vi "Pressure_2_R1.vi"() -> ()   [LabVIEW 2020]
uses:
  Support/Controls/Cmd_Mouse Popup.ctl
  Support/Controls/Clst_Initialize Input.ctl
  Support/Controls/Cmd_Var Data IO.ctl
  Variables/Global_Cal Info.vi
panel:
  in  "Measured_ADJ":string[][](table) caption="Measured (조정후)"
  in  "입력전압":dbl=10.0 caption="(V)"
  in  "정격출력":dbl
  in  "최소출력":dbl
  in  "출력단위":string(combo)="V"
  out "최소용량":string
  out "분동조합":string[][](table)
  out "Form":string[][](table)
  in  "교정방법":string(combo)="기본교정"
  out "Resolution":string[][](table) caption="Spec"
  in  "Spec 변경":bool
  in  "Random":bool
  out "Spec":string[][](table)
  out "제목":string
  out "에러 출력":errorcluster
  out "Condition":string[][](table)
  out "최소눈금":string
  out "단위":string
  out "최대용량":string
  in  "Measured":string[][](table)
  out "Load?":bool
  # "※ 압력기준기 복수 선택 시 분동식 압력계\n    우선 적용됨."
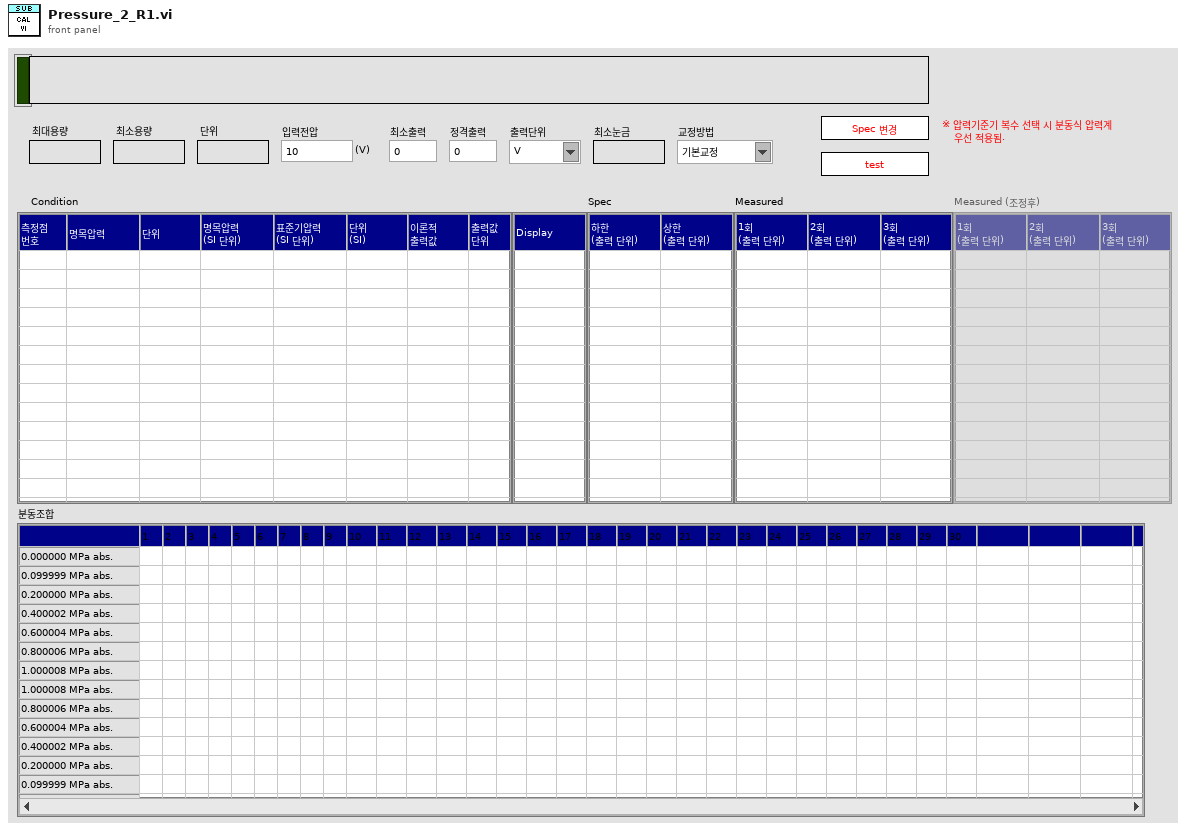
[diagram p1: front panel]
types:
  T1 = typedef "Cmd_Mouse Popup.ctl" = enum16{"활성화", "메뉴선택"}
  T2 = cluster{"Shift":bool, "Ctrl":bool, "Alt":bool, "Cmd":bool, "Opt":bool}
  T3 = typedef "Clst_Initialize Input.ctl" = cluster{"Initialize 1":cluster{"Condition":refnum<vi>[], "Spec":refnum<vi>[], "Measured":refnum<vi>[], "Resolution":refnum<vi>[], "Func_ext":string, "제목":refnum<vi>, "Measured_ADJ":refnum<vi>[]}, "Initialize 2":cluster{"문자열":refnum<vi>[], "콤보박스":refnum<vi>[], "링":refnum<vi>[], "열거형":refnum<vi>[], "테이블":refnum<vi>[], "여러열":refnum<vi>[], "디지털(DBL)":refnum<vi>[], "3D string":refnum<vi>[], "ctrl":refnum<vi>[], "boolean":refnum<vi>[]}}
  T4 = typedef "Cmd_Var Data IO.ctl" = enum16{"Condition", "Condition Default", "Condition_Temp", "Resolution", "Resolution Default", "Resolution Old", "Spec", "Spec Default", "Spec Old", "Spec Temp", "Result", "Result2", "Result3", "Result_Temp", "Result_ADJ", "Result_ADJ2", "STD1", "STD2", "STD3", "STD4", "STD5", "STD Temp", "CMC", "CMC Default"}
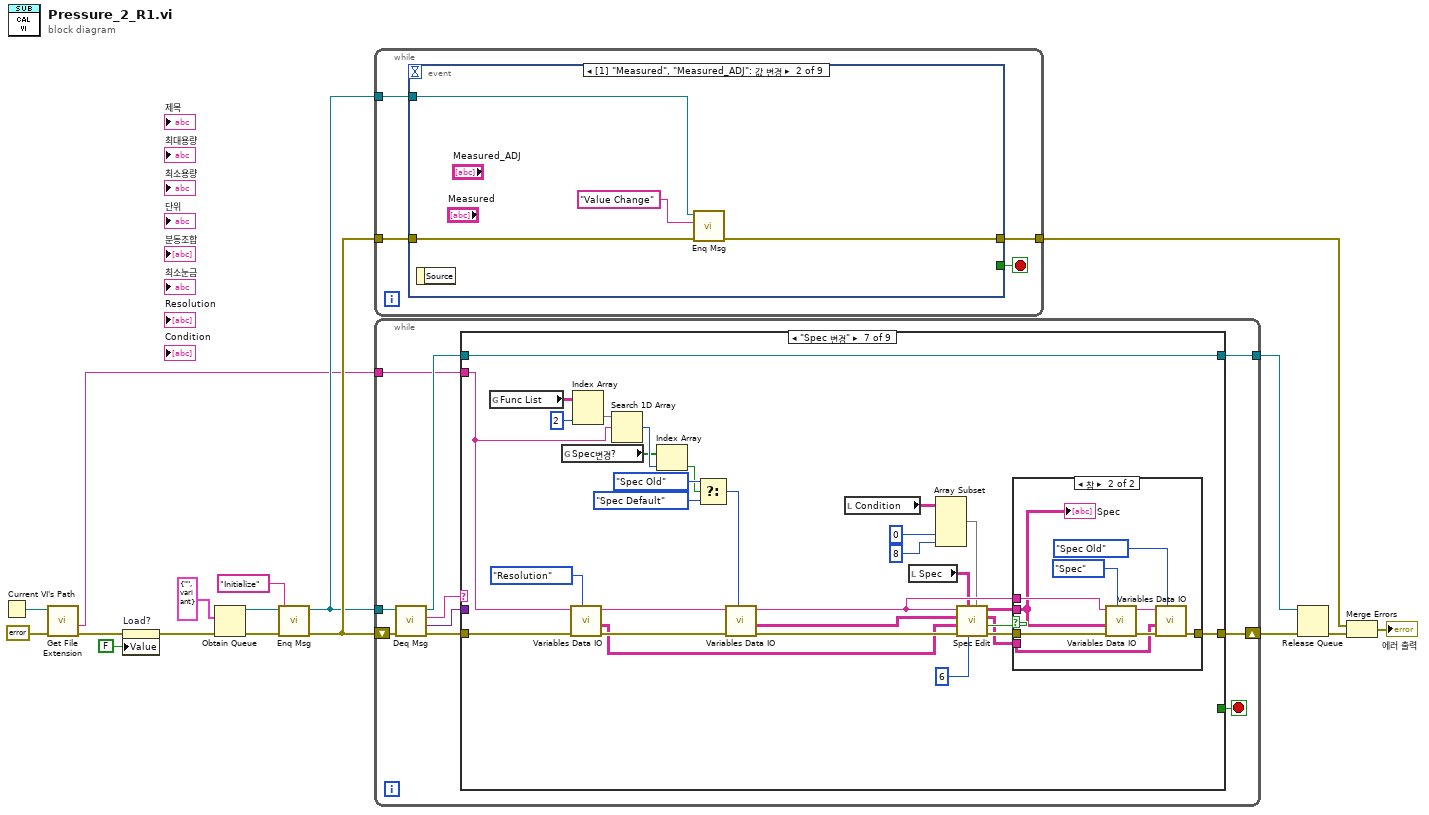
[diagram p0: block diagram]
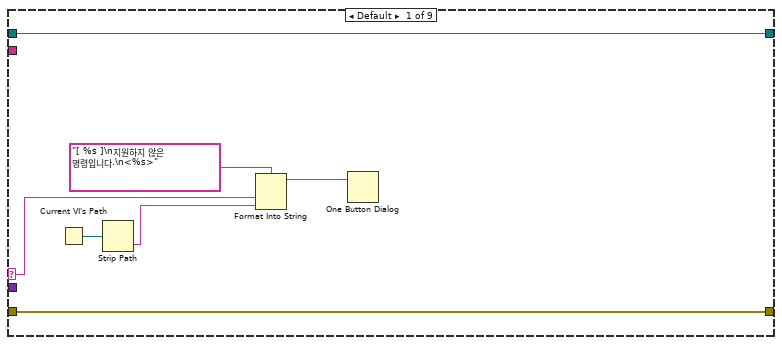
[diagram p2: hidden frame]
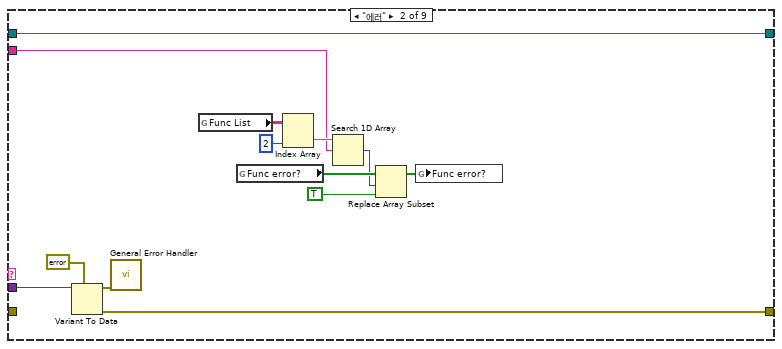
[diagram p3: hidden frame]
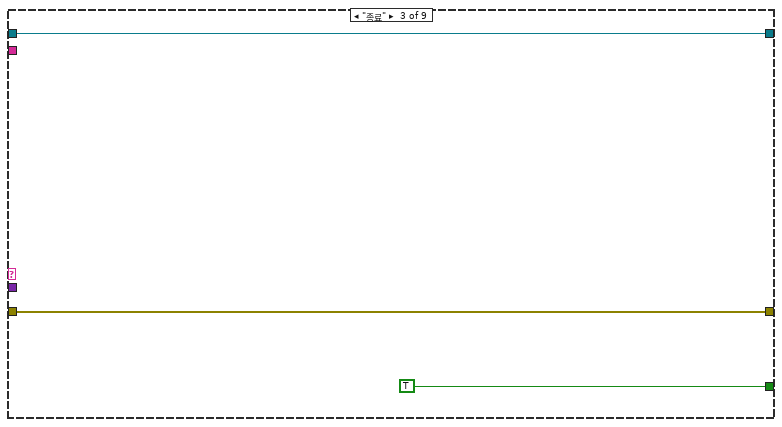
[diagram p4: hidden frame]
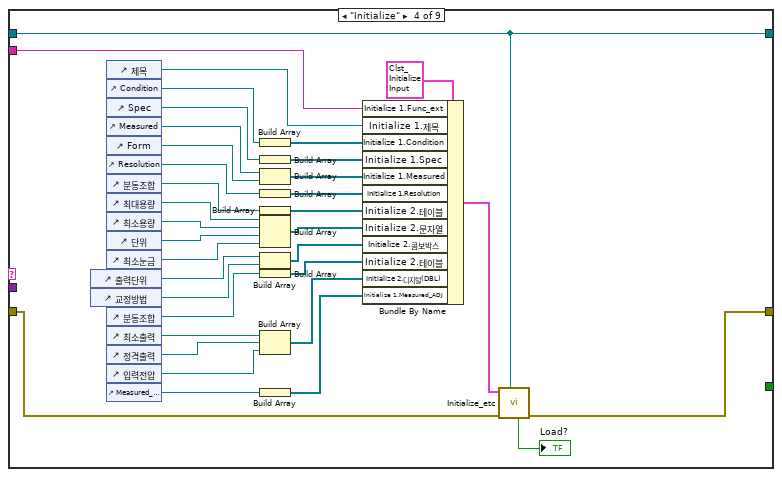
[diagram p5: hidden frame]
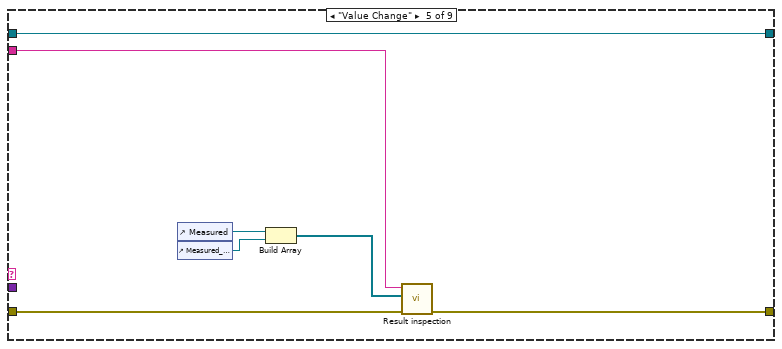
[diagram p6: hidden frame]
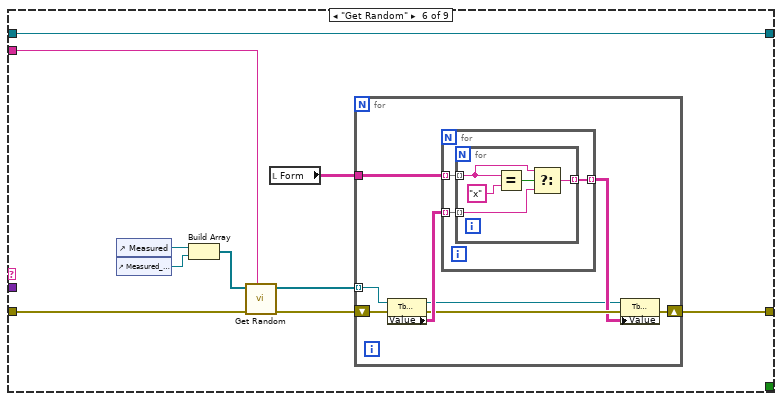
[diagram p7: hidden frame]
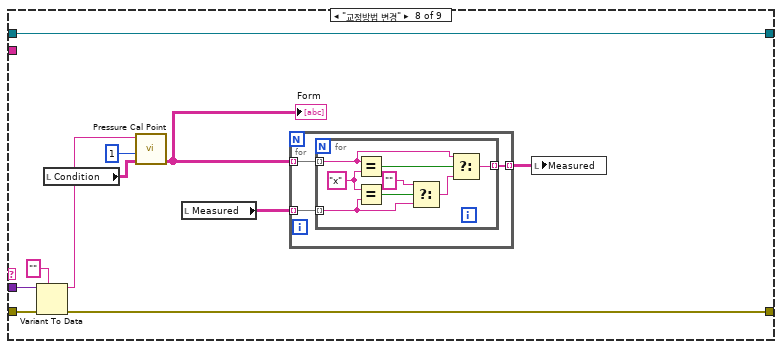
[diagram p9: hidden frame]
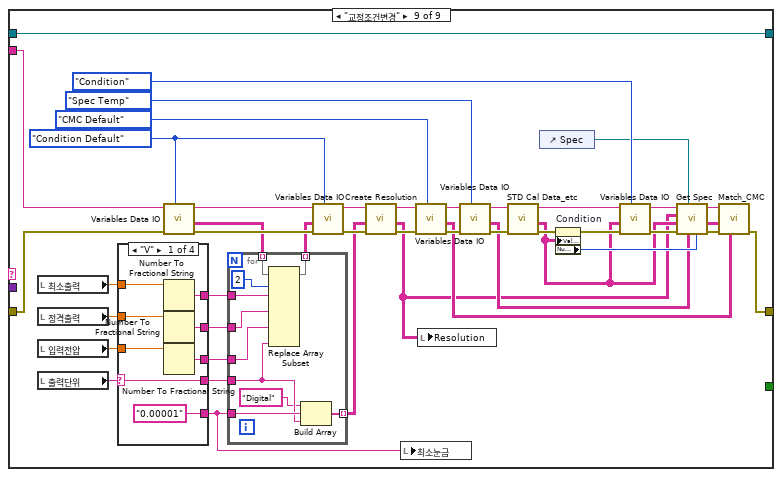
[diagram p10: hidden frame]
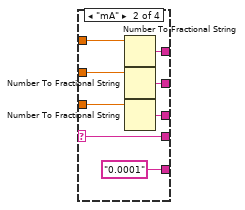
[diagram p11: hidden frame]
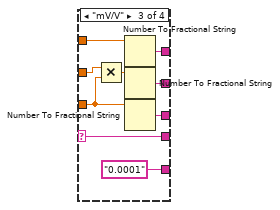
[diagram p12: hidden frame]
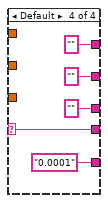
[diagram p13: hidden frame]
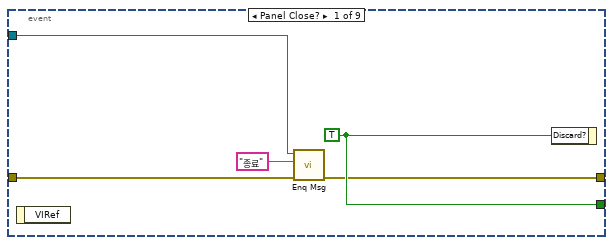
[diagram p14: hidden frame]
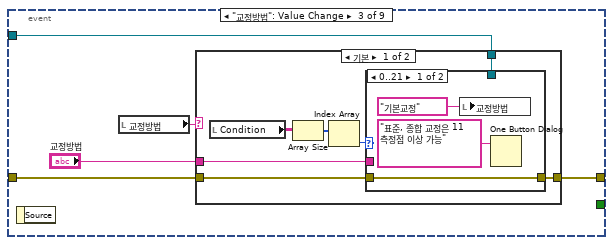
[diagram p15: hidden frame]
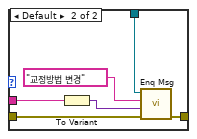
[diagram p16: hidden frame]
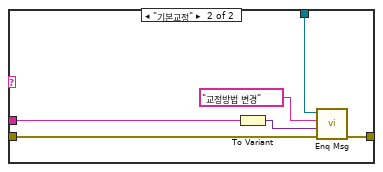
[diagram p17: hidden frame]
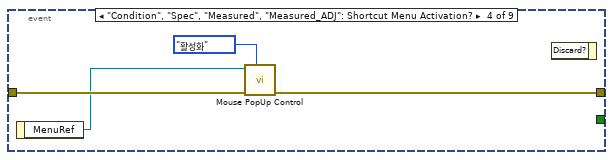
[diagram p18: hidden frame]
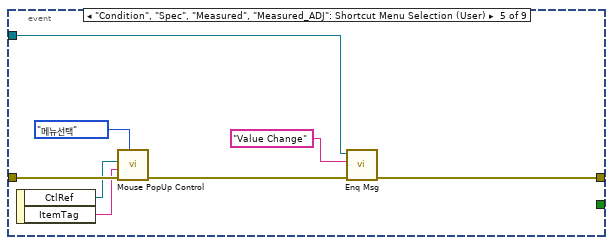
[diagram p19: hidden frame]
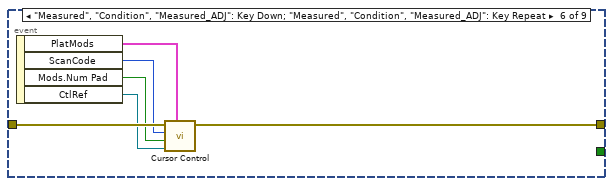
[diagram p20: hidden frame]
diagram:
  n1 = Current VI's Path() -> (path=w5:path)
  n2 = call <vilib>:"Get File Extension.vi"("error in (no error)"=errorcluster {"status"=FALSE, "code"=0, "source"=""} ("에러 상수"), "file"=w5) -> ("error out"=w3:errorcluster, "filename without extension"=w4:string)  [unwired: 5 in, 3 out]
  n3 = property on="Load?" class="Bool (엄격한)"(error in=w3, "Value"=FALSE ("Load?")) -> (error out=w2:errorcluster)  [unwired: 1 in, 1 out]
  n4 = Obtain Queue(element data type=cluster{"메세지":string, "값":variant} {"메세지"="", "값"=variant} ("Message Cluster"), error in (no error)=w2) -> (queue out=w14:refnum<queue>, error out=w16:errorcluster)  [unwired: 3 in, 1 out]
  n5 = call "Enq Msg.vi"("에러 입력(에러 없음)"=w16, "메세지"="Initialize", "큐 입력"=w14) -> ("에러 출력"=w15:errorcluster, "큐 출력"=w12:refnum<queue>)  [unwired: 7 in]
  n6 = while {
    tunnel: w15 -> [w19]
    tunnel: w12 -> [w20]
    tunnel: [w18] -> w9
    stop <- w21 stop-if-true
    n7 = event shown="[1] \"Measured\", \"Measured_ADJ\": 값 변경" {
      selector: _ -> [_ _ _ _ _ _ _ _ _]
      dyn-events: _ -> [_ _ _ _ _ _ _ _ _]
      timeout: _ -> [_ _ _ _ _ _ _ _ _]
      tunnel: [w26 _ _ _ _ _ _ _ _] -> w21
      tunnel: w20 -> [w24 w29 w32 _ w64 _ w77 w83 w87]
      tunnel: w19 -> [w25 w30 w34 w60 w68 w75 w78 w85 w89]
      tunnel: [w22 w28 w35 w59 w63 w74 w76 w84 w88] -> w18
      event Panel Close? {
        w26 = TRUE ("버림?")
        n8 = event-data() -> ()  [unwired: 1 in, 1 out]
        n9 = call "Enq Msg.vi"("에러 입력(에러 없음)"=w25, "메세지"="종료", "큐 입력"=w24) -> ("에러 출력"=w22:errorcluster)  [unwired: 7 in, 1 out]
        n10 = event-data("Discard?"=w26) -> ()  [unwired: 1 in, 1 out]
      }
      event "Measured", "Measured_ADJ": Value Change {
        n11 = event-data() -> ()  [unwired: 1 in, 1 out]
        n12 = call "Enq Msg.vi"("에러 입력(에러 없음)"=w30, "메세지"="Value Change", "큐 입력"=w29) -> ("에러 출력"=w28:errorcluster)  [unwired: 7 in, 1 out]
      }
      event "교정방법": Value Change {
        n13 = event-data() -> ()  [unwired: 1 in, 1 out]
        n14 = local read "교정방법"() -> (w31:string)
        n15 = case shown="기본" w31 {
          tunnel: w34 -> [w42 w57]
          tunnel: w32 -> [w41 w56]
          tunnel: [w40 w55] -> w35
          tunnel: "교정방법" -> [w39 w54]
          frame Default {
            n16 = local read "Condition"() -> (w36:string[][])
            n17 = Array Size(array=w36) -> (size(s)=w38:i32[])
            n18 = Index Array(array=w38) -> (element=w37:i32)  [unwired: 1 in]
            n19 = case shown="0..21" w37 {
              tunnel: w42 -> [w45 w51]
              tunnel: w41 -> [_ w50]
              tunnel: [w45 w48] -> w40
              tunnel: w39 -> [_ w46]
              frame 0..21 {
                n20 = local write "교정방법"("기본교정" ("교정방법")) -> ()
                n21 = One Button Dialog(message="표준, 종합 교정은 11 측정점 이상 가능" ("메시지")) -> ()  [unwired: 1 in, 1 out]
              }
              frame Default {
                n22 = To Variant(anything=w46) -> (Variant=w47:variant)
                n23 = call "Enq Msg.vi"("에러 입력(에러 없음)"=w51, "값"=w47, "메세지"="교정방법 변경", "큐 입력"=w50) -> ("에러 출력"=w48:errorcluster)  [unwired: 6 in, 1 out]
              }
            }
          }
          frame "기본교정" {
            n24 = To Variant(anything=w54) -> (Variant=w52:variant)
            n25 = call "Enq Msg.vi"("에러 입력(에러 없음)"=w57, "값"=w52, "메세지"="교정방법 변경", "큐 입력"=w56) -> ("에러 출력"=w55:errorcluster)  [unwired: 6 in, 1 out]
          }
        }
      }
      event "Condition", "Spec", "Measured", "Measured_ADJ": Shortcut Menu Activation? {
        n26 = event-data() -> ("MenuRef"=w58:refnum<k9>)  [unwired: 1 in]
        n27 = call "Mouse PopUp Control.vi"("type"=Cmd_Mouse_Popup."활성화", "error in"=w60, "메뉴 참조"=w58) -> ("error out"=w59:errorcluster)  [unwired: 8 in]
        n28 = event-data() -> ()  [unwired: 2 in, 1 out]
      }
      event "Condition", "Spec", "Measured", "Measured_ADJ": Shortcut Menu Selection (User) {
        n29 = event-data() -> ("CtlRef"=w66:refnum<vi>, "ItemTag"=w67:string)  [unwired: 1 in]
        n30 = call "Mouse PopUp Control.vi"("type"=Cmd_Mouse_Popup."메뉴선택", "error in"=w68, "아이템 태그"=w67, "Tbl 참조 번호"=w66) -> ("error out"=w65:errorcluster)  [unwired: 7 in]
        n31 = call "Enq Msg.vi"("에러 입력(에러 없음)"=w65, "메세지"="Value Change", "큐 입력"=w64) -> ("에러 출력"=w63:errorcluster)  [unwired: 7 in, 1 out]
      }
      event "Measured", "Condition", "Measured_ADJ": Key Down; "Measured", "Condition", "Measured_ADJ": Key Repeat {
        n32 = event-data() -> ("PlatMods"=w70:T2, "ScanCode"=w73:i16, "Mods.Num Pad"=w72:bool, "CtlRef"=w71:refnum<vi>)  [unwired: 1 in]
        n33 = call "Cursor Control.vi"("플랫폼 조합키"=w70, "참조"=w71, "Num Pad"=w72, "ScanCode"=w73, "error in"=w75) -> ("error out"=w74:errorcluster)  [unwired: 5 in, 1 out]
      }
      event "Random": Value Change {
        n34 = event-data() -> ()  [unwired: 1 in, 1 out]
        n35 = call "Enq Msg.vi"("에러 입력(에러 없음)"=w78, "메세지"="Get Random", "큐 입력"=w77) -> ("에러 출력"=w80:errorcluster, "큐 출력"=w81:refnum<queue>)  [unwired: 7 in]
        n36 = call "Enq Msg.vi"("에러 입력(에러 없음)"=w80, "메세지"="Value Change", "큐 입력"=w81) -> ("에러 출력"=w76:errorcluster)  [unwired: 7 in, 1 out]
      }
      event "Spec 변경": Value Change {
        n37 = event-data() -> ()  [unwired: 1 in, 1 out]
        n38 = call "Enq Msg.vi"("에러 입력(에러 없음)"=w85, "메세지"="Spec 변경", "큐 입력"=w83) -> ("에러 출력"=w84:errorcluster)  [unwired: 7 in, 1 out]
      }
      event "정격출력", "최소출력", "입력전압", "출력단위": Value Change {
        n39 = event-data() -> ()  [unwired: 1 in, 2 out]
        n40 = call "Enq Msg.vi"("에러 입력(에러 없음)"=w89, "메세지"="교정조건변경", "큐 입력"=w87) -> ("에러 출력"=w88:errorcluster)  [unwired: 7 in, 1 out]
      }
    }
  }
  n41 = while {
    shift-right: [w100] -> w11
    shift-left: w15 -> [w99]
    tunnel: w12 -> [w97]
    tunnel: [w92] -> w10
    tunnel: w4 -> [w91]
    stop <- w93 stop-if-true
    n42 = call "Deq Msg.vi"("에러 입력(에러 없음)"=w99, "큐 입력"=w97) -> ("에러 출력"=w98:errorcluster, "값"=w94:variant, "메세지"=w96:string, "큐 출력"=w95:refnum<queue>)  [unwired: 6 in]
    n43 = case shown="\"Spec 변경\"" w96 {
      selector: w96 -> [w103 _ _ _ _ _ _ _ _]
      tunnel: w98 -> [w107 _ w123 w143 w162 w173 w215 w239 w278]
      tunnel: [w107 w117 w123 w125 w164 w168 w219 w238 w290] -> w100
      tunnel: w95 -> [w106 w116 w121 w144 w165 w175 w221 w242 w297]
      tunnel: w94 -> [_ w118 _ _ _ _ _ w240 _]
      tunnel: [_ _ TRUE ("버림?") _ _ _ _ _ _] -> w93
      tunnel: [w106 w116 w121 w144 w165 w175 w221 w242 w297] -> w92
      tunnel: w91 -> [_ w108 _ w135 w163 w171 w197 _ w279]
      frame Default {
        n44 = Current VI's Path() -> (path=w102:path)
        n45 = Strip Path(path=w102) -> (name=w101:string)  [unwired: 1 out]
        n46 = Format Into String(format string="[ %s ]\n지원하지 않은 명령입니다.\n<%s>" ("메시지"), w103, w101) -> (resulting string=w104:string)  [unwired: 2 in, 1 out]
        n47 = One Button Dialog(message=w104) -> ()  [unwired: 1 in, 1 out]
      }
      frame "에러" {
        n48 = Variant To Data(type=errorcluster {"status"=FALSE, "code"=0, "source"=""} ("에러 출력"), Variant=w118) -> (data=w120:errorcluster, error out=w117:errorcluster)  [unwired: 1 in]
        n49 = call <vilib>:"General Error Handler.vi"("error in (no error)"=w120) -> ()  [unwired: 10 in, 5 out]
        n50 = global read "Global_Cal Info.vi" "Func List"() -> (w114:string[][])
        n51 = global read "Global_Cal Info.vi" "Func error?"() -> (w111:bool[])
        n52 = Index Array(array=w114, index (col)=2 ("비활성화된 인덱스 (열)")) -> (element=w113:string[])  [unwired: 1 in]
        n53 = Search 1D Array(1D array=w113, element=w108) -> (index of element=w110:i32)  [unwired: 1 in]
        n54 = Replace Array Subset(array=w111, new element=TRUE ("새 원소/부분배열"), index=w110) -> (w109:bool[])
        n55 = global write "Global_Cal Info.vi" "Func error?"(w109) -> ()
      }
      frame "종료" {
      }
      frame "Initialize" {
        n56 = control-ref of="출력단위"() -> (w132:refnum<vi>)
        n57 = control-ref of="교정방법"() -> (w139:refnum<vi>)
        n58 = control-ref of="제목"() -> (w149:refnum<vi>)
        n59 = control-ref of="Condition"() -> (w156:refnum<vi>)
        n60 = control-ref of="Spec"() -> (w146:refnum<vi>)
        n61 = control-ref of="Measured"() -> (w153:refnum<vi>)
        n62 = control-ref of="Form"() -> (w137:refnum<vi>)
        n63 = control-ref of="Resolution"() -> (w141:refnum<vi>)
        n64 = control-ref of="분동조합"() -> (w142:refnum<vi>)
        n65 = control-ref of="최대용량"() -> (w148:refnum<vi>)
        n66 = control-ref of="최소용량"() -> (w134:refnum<vi>)
        n67 = control-ref of="단위"() -> (w147:refnum<vi>)
        n68 = control-ref of="최소눈금"() -> (w133:refnum<vi>)
        n69 = control-ref of="분동조합"() -> (w136:refnum<vi>)
        n70 = control-ref of="최소출력"() -> (w131:refnum<vi>)
        n71 = control-ref of="정격출력"() -> (w130:refnum<vi>)
        n72 = control-ref of="입력전압"() -> (w129:refnum<vi>)
        n73 = control-ref of="Measured_ADJ"() -> (w127:refnum<vi>)
        n74 = Build Array(w156) -> (w155:refnum<vi>[])
        n75 = Build Array(w146) -> (w145:refnum<vi>[])
        n76 = Build Array(w153, w137) -> (w154:refnum<vi>[])
        n77 = Build Array(w141) -> (w140:refnum<vi>[])
        n78 = Build Array(w142) -> (w152:refnum<vi>[])
        n79 = Build Array(w148, w134, w147, w133) -> (w151:refnum<vi>[])
        n80 = Build Array(w132, w139) -> (w150:refnum<vi>[])
        n81 = Build Array(w136) -> (w138:refnum<vi>[])
        n82 = Build Array(w131, w130, w129) -> (w128:refnum<vi>[])
        n83 = Build Array(w127) -> (w126:refnum<vi>[])
        n84 = Bundle By Name(cluster=T3 {"Initialize 1"={"Condition"=[], "Spec"=[], "Measured"=[], "Resolution"=[], "Func_ext"="", "제목"=refnum, "Measured_ADJ"=[]}, "Initialize 2"={"문자열"=[], "콤보박스"=[], "링"=[], "열거형"=[], "테이블"=[], "여러열"=[], "디지털(DBL)"=[], "3D string"=[], "ctrl"=[], "boolean"=[]}} ("입력 클러스터"), "Initialize 1.Func_ext"=w135, "Initialize 1.제목"=w149, "Initialize 1.Condition"=w155, "Initialize 1.Spec"=w145, "Initialize 1.Measured"=w154, "Initialize 1.Resolution"=w140, "Initialize 2.테이블"=w152, "Initialize 2.문자열"=w151, "Initialize 2.콤보박스"=w150, "Initialize 2.테이블"=w138, "Initialize 2.디지털(DBL)"=w128, "Initialize 1.Measured_ADJ"=w126) -> (w157:T3)
        n85 = call "Initialize_etc.vi"("큐 입력"=w144, "error in"=w143, "입력 클러스터"=w157) -> ("error out"=w125:errorcluster, "Load?"=→"Load?":bool)  [unwired: 6 in, 1 out]
      }
      frame "Value Change" {
        n86 = control-ref of="Measured"() -> (w161:refnum<vi>)
        n87 = control-ref of="Measured_ADJ"() -> (w159:refnum<vi>)
        n88 = Build Array(w161, w159) -> (w160:refnum<vi>[])
        n89 = call "Result inspection.vi"("error in"=w162, "Ref. Data (Inspection)"=w160, "Func ext"=w163) -> ("error out"=w164:errorcluster)  [unwired: 5 in, 3 out]
      }
      frame "Get Random" {
        n90 = control-ref of="Measured"() -> (w172:refnum<vi>)
        n91 = control-ref of="Measured_ADJ"() -> (w170:refnum<vi>)
        n92 = Build Array(w172, w170) -> (w174:refnum<vi>[])
        n93 = call "Get Random.vi"("Func_Ext"=w171, "에러 입력"=w173, "Meas"=w174) -> ("에러 출력"=w169:errorcluster, "Meas out"=w167:refnum<vi>[])  [unwired: 7 in]
        n94 = local read "Form"() -> (w166:string[][])
        n95 = for {
          tunnel: w166 -> [w182]
          shift-right: [w179] -> w168
          shift-left: w169 -> [w183]
          tunnel: w167 -> [w176] mode=indexing
          n96 = property on="프로퍼티 노드" class="Tbl (엄격한)"(reference=w176, error in=w183) -> (reference out=w177:refnum<vi>, error out=w180:errorcluster, "Value"=w181:string[][])
          n97 = for {
            tunnel: w182 -> [w186] mode=indexing
            tunnel: w181 -> [w185] mode=indexing
            tunnel: [w184] -> w178 mode=indexing
            n98 = for {
              tunnel: w186 -> [w189] mode=indexing
              tunnel: w185 -> [w188] mode=indexing
              tunnel: [w187] -> w184 mode=indexing
              n99 = Equal?(x=w189, y="ⅹ") -> (x = y?=w190:bool)
              n100 = Select(t=w189, s=w190, f=w188) -> (s? t:f=w187:string)
            }
          }
          n101 = property on="프로퍼티 노드" class="Tbl (엄격한)"(reference=w177, error in=w180, "Value"=w178) -> (error out=w179:errorcluster)  [unwired: 1 out]
        }
      }
      frame "Spec 변경" {
        n102 = global read "Global_Cal Info.vi" "Func List"() -> (w202:string[][])
        n103 = global read "Global_Cal Info.vi" "Spec변경?"() -> (w198:bool[])
        n104 = call "Variables Data IO.vi"("Select"=Cmd_Var_Data_IO."Resolution", "error in"=w215, "Func_ext"=w197) -> ("error out"=w214:errorcluster, "Data Out"=w208:string[][], "Func_ext Out"=w213:string)  [unwired: 6 in]
        n105 = Index Array(array=w202, index (col)=2 ("비활성화된 인덱스 (열)")) -> (element=w200:string[])  [unwired: 1 in]
        n106 = Search 1D Array(1D array=w200, element=w197) -> (index of element=w199:i32)  [unwired: 1 in]
        n107 = Index Array(array=w198, index=w199) -> (element=w203:bool)
        n108 = Select(t=Cmd_Var_Data_IO."Spec Old" ("Select"), s=w203, f=Cmd_Var_Data_IO."Spec Default" ("Select")) -> (s? t:f=w196:T4)
        n109 = call "Variables Data IO.vi"("Select"=w196, "error in"=w214, "Func_ext"=w213) -> ("error out"=w216:errorcluster, "Data Out"=w207:string[][], "Func_ext Out"=w209:string)  [unwired: 6 in]
        n110 = local read "Condition"() -> (w195:string[][])
        n111 = local read "Spec"() -> (w206:string[][])
        n112 = Array Subset(array=w195, index (col)=0 ("인덱스"), length (col)=8 ("길이")) -> (w192:string[][])  [unwired: 2 in]
        n113 = call "Spec Edit.vi"("Condition"=w192, "열번호(기준값)"=6 ("기준열(0)"), "Spec Value"=w206, "에러 입력(에러 없음)"=w216, "Resolution"=w208, "Spec Default"=w207, "Func_ext"=w209) -> ("에러 출력"=w220:errorcluster, "변경?"=w217:bool, "Spec Default out"=w211:string[][], "Spec 출력"=w218:string[][])  [unwired: 1 in]
        n114 = case shown="참" w217 {
          tunnel: w220 -> [w222 w230]
          tunnel: [w222 w226] -> w219
          tunnel: w218 -> [_ w228]
          tunnel: w209 -> [_ w229]
          tunnel: w211 -> [_ w224]
          frame False {
          }
          frame True {
            n115 = call "Variables Data IO.vi"("Select"=Cmd_Var_Data_IO."Spec", "error in"=w230, "Data In"=w228, "Func_ext"=w229) -> ("error out"=w227:errorcluster, "Func_ext Out"=w225:string)  [unwired: 5 in, 1 out]
            n116 = call "Variables Data IO.vi"("Select"=Cmd_Var_Data_IO."Spec Old", "error in"=w227, "Data In"=w224, "Func_ext"=w225) -> ("error out"=w226:errorcluster)  [unwired: 5 in, 2 out]
            "Spec" <- w228
          }
        }
      }
      frame "교정방법 변경" {
        n117 = Variant To Data(error in=w239, type="", Variant=w240) -> (data=w235:string, error out=w238:errorcluster)
        n118 = local read "Condition"() -> (w234:string[][])
        n119 = call "Pressure Cal Point.vi"("Condition"=w234, "인덱스 (열)"=1, "교정방법"=w235) -> ("배열"=w232:string[][])  [unwired: 5 in, 3 out]
        "Form" <- w232
        n120 = local read "Measured"() -> (w237:string[][])
        n121 = for {
          tunnel: w232 -> [w245] mode=indexing
          tunnel: w237 -> [w244] mode=indexing
          tunnel: [w243] -> w236 mode=indexing
          n122 = for {
            tunnel: w245 -> [w252] mode=indexing
            tunnel: w244 -> [w248] mode=indexing
            tunnel: [w246] -> w243 mode=indexing
            w251 = "ⅹ"
            n123 = Equal?(x=w252, y=w251) -> (x = y?=w253:bool)
            n124 = Equal?(x=w251, y=w248) -> (x = y?=w250:bool)
            n125 = Select(t="", s=w250, f=w248) -> (s? t:f=w247:string)
            n126 = Select(t=w252, s=w253, f=w247) -> (s? t:f=w246:string)
          }
        }
        n127 = local write "Measured"(w236) -> ()
      }
      frame "교정조건변경" {
        w275 = Cmd_Var_Data_IO."Condition Default" ("Select")
        n128 = local read "최소출력"() -> (w272:dbl)
        n129 = local read "정격출력"() -> (w271:dbl)
        n130 = local read "입력전압"() -> (w270:dbl)
        n131 = local read "출력단위"() -> (w269:string)
        n132 = case shown="\"V\"" w269 {
          selector: w269 -> [w303 w311 w321 w326]
          tunnel: ["0.00001" "0.0001" "0.0001" "0.0001"] -> w259
          tunnel: w272 -> [w304 w312 w317 _]
          tunnel: w271 -> [w301 w309 w314 _]
          tunnel: w270 -> [w300 w308 w316 _]
          tunnel: [w303 w311 w321 w326] -> w268
          tunnel: [w302 w310 w320 ""] -> w265
          tunnel: [w299 w307 w319 ""] -> w266
          tunnel: [w298 w306 w318 ""] -> w267
          frame "V" {
            n133 = Number To Fractional String(number=w304) -> (F-format string=w302:string)  [unwired: 3 in]
            n134 = Number To Fractional String(number=w301) -> (F-format string=w299:string)  [unwired: 3 in]
            n135 = Number To Fractional String(number=w300) -> (F-format string=w298:string)  [unwired: 3 in]
          }
          frame "mA" {
            n136 = Number To Fractional String(number=w312) -> (F-format string=w310:string)  [unwired: 3 in]
            n137 = Number To Fractional String(number=w309) -> (F-format string=w307:string)  [unwired: 3 in]
            n138 = Number To Fractional String(number=w308) -> (F-format string=w306:string)  [unwired: 3 in]
          }
          frame "mV/V" {
            n139 = Multiply(x=w314, y=w316) -> (x*y=w315:dbl)
            n140 = Number To Fractional String(number=w317) -> (F-format string=w320:string)  [unwired: 3 in]
            n141 = Number To Fractional String(number=w315) -> (F-format string=w319:string)  [unwired: 3 in]
            n142 = Number To Fractional String(number=w316) -> (F-format string=w318:string)  [unwired: 3 in]
          }
          frame Default {
          }
        }
        n143 = call "Variables Data IO.vi"("Select"=w275, "error in"=w278, "Func_ext"=w279) -> ("error out"=w277:errorcluster, "Data Out"=w274:string[][], "Func_ext Out"=w276:string)  [unwired: 6 in]
        n144 = for {
          tunnel: w274 -> [w337] mode=indexing
          tunnel: [w336] -> w273 mode=indexing
          tunnel: w268 -> [w330]
          tunnel: w267 -> [w334]
          tunnel: w266 -> [w333]
          tunnel: w265 -> [w332]
          tunnel: w259 -> [w331]
          tunnel: [w328] -> w260 mode=indexing
          n145 = Replace Array Subset(array=w337, new element #1=w332, index #1=2 ("인덱스"), new element #2=w333, new element #3=w334, new element #4=w330) -> (w336:string[])  [unwired: 3 in]
          n146 = Build Array("Digital" ("원소"), w331, w330) -> (w328:string[])
        }
        n147 = call "Variables Data IO.vi"("Select"=w275, "error in"=w277, "Data In"=w273, "Func_ext"=w276) -> ("error out"=w264:errorcluster, "Func_ext Out"=w262:string)  [unwired: 5 in, 1 out]
        n148 = call "Create Resolution.vi"("에러 입력(에러 없음)"=w264, "Resolution"=w260, "Func_ext"=w262) -> ("에러 출력"=w263:errorcluster, "Resolution Out"=w255:string[][], "Func_ext 출력"=w261:string)  [unwired: 6 in]
        n149 = local write "최소눈금"(w259) -> ()
        n150 = call "Variables Data IO.vi"("Select"=Cmd_Var_Data_IO."CMC Default", "error in"=w263, "Func_ext"=w261) -> ("error out"=w286:errorcluster, "Data Out"=w283:string[][], "Func_ext Out"=w285:string)  [unwired: 6 in]
        n151 = local write "Resolution"(w255) -> ()
        n152 = call "Variables Data IO.vi"("Select"=Cmd_Var_Data_IO."Spec Temp", "error in"=w286, "Func_ext"=w285) -> ("error out"=w289:errorcluster, "Data Out"=w257:string[][], "Func_ext Out"=w288:string)  [unwired: 6 in]
        n153 = call "STD Cal Data_etc.vi"("error in"=w289, "Func_ext"=w288) -> ("error out"=w281:errorcluster, "Data Out"=w256:string[][], "Func_ext Out"=w293:string)  [unwired: 5 in, 2 out]
        n154 = control-ref of="Spec"() -> (w282:refnum<vi>)
        n155 = property on="Condition" class="Tbl (엄격한)"(error in=w281, "Value"=w256) -> (error out=w280:errorcluster, "Number of Rows"=w258:u32)  [unwired: 1 in, 1 out]
        n156 = call "Variables Data IO.vi"("Select"=Cmd_Var_Data_IO."Condition", "error in"=w280, "Data In"=w256, "Func_ext"=w293) -> ("error out"=w296:errorcluster, "Func_ext Out"=w254:string)  [unwired: 5 in, 1 out]
        n157 = call "Get Spec.vi"("NumRows"=w258, "Spec in"=w257, "Spec Ref."=w282, "error in"=w296, "Condition in"=w256, "Resolution in"=w255, "Func_ext"=w254) -> ("error out"=w291:errorcluster, "Data Out"=w295:string[][], "Func_ext Out"=w292:string)  [unwired: 2 out]
        n158 = call "Match_CMC.vi"("CMC IN"=w283, "error in"=w291, "Condition IN"=w295, "Func_ext"=w292) -> ("error out"=w290:errorcluster)  [unwired: 4 in, 3 out]
      }
    }
  }
  n159 = Release Queue(queue=w10, error in (no error)=w11) -> (error out=w8:errorcluster)  [unwired: 1 in, 2 out]
  n160 = Merge Errors(w9, w8) -> (→"에러 출력":errorcluster)
